vi "Get Session ID.vi"(11 "WelcomeHandler MsgPack in":refnum<class "WelcomeHandler MsgPack.lvclass">) -> (2 "Session ID":u64, 3 "WelcomeHandler MsgPack out":refnum<class "WelcomeHandler MsgPack.lvclass">)   [LabVIEW 2020, in "wamplv.lvlib" / "WelcomeHandler MsgPack.lvclass"]
uses:
  WelcomeHandler MsgPack.lvclass
  WelcomeHandler MsgPack.lvclass/WelcomeHandler MsgPack.ctl
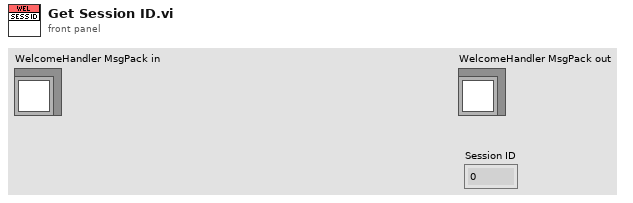
[diagram p1: front panel]
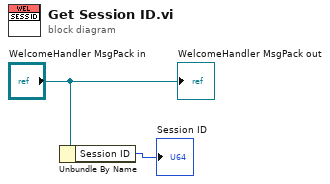
[diagram p0: block diagram]
diagram:
  n1 = Unbundle By Name("WelcomeHandler MsgPack in") -> ("Session ID"=→"Session ID":u64)
  "WelcomeHandler MsgPack out" <- "WelcomeHandler MsgPack in"
